vi "UE9 4-Channel Frequency Output.vi"(8 "error in":errorcluster, 10 "Timer0 Frequency [Hz]":dbl=1000.0 format="%.1f") -> (0 "error out":errorcluster, 2 "Actual Frequency 0":dbl format="%.1f")   [LabVIEW 2021]
panel:
  in  "Case Constant\n(See Context Help)":bool
  out "FreqDivisor3":u8
  out "FreqDivisor2":u8
  out "FreqDivisor1":u8
  out "FreqDivisor0":u8
  out "Actual Frequency 3":dbl format="%.1f"
  out "Actual Frequency 2":dbl format="%.1f"
  out "Actual Frequency 1":dbl format="%.1f"
  in  "Timer3 Frequency [Hz]":dbl=4000.0 format="%.1f"
  in  "Timer2 Frequency [Hz]":dbl=3000.0 format="%.1f"
  in  "Timer1 Frequency [Hz]":dbl=2000.0 format="%.1f"
  in  "FirstFound":bool=TRUE
  in  "Address":string="1"
  in  "ConnectionType":u16(ring) items=["LJ_ctUSB", "LJ_ctETHERNET"]
  in  "# of frequency outputs to enable":u32=4
  out "TimerClockDivisor":u8
  out "TimerClockConfig":string
  out "Error Message":string
  # "Demonstrates 4 channels of frequency output on FIO0-FIO3.\nAssumes Control power level is at the default level of \"High\" (Control firmware 1.08 or higher).\nA simple algorithm decides the clock settings to get the desired Timer0 frequency.  Then the\nfrequency divisor value is adjusted, as much as possible, to get the frequencies specified for\nother channels.  Because of these simple algorithms, best results will most likely occur if Timer0 is\nthe lowest frequency of the 4."
  # "Clock configuration determined\nby first channel."
  # "24 MHz max, 5.7 Hz min"
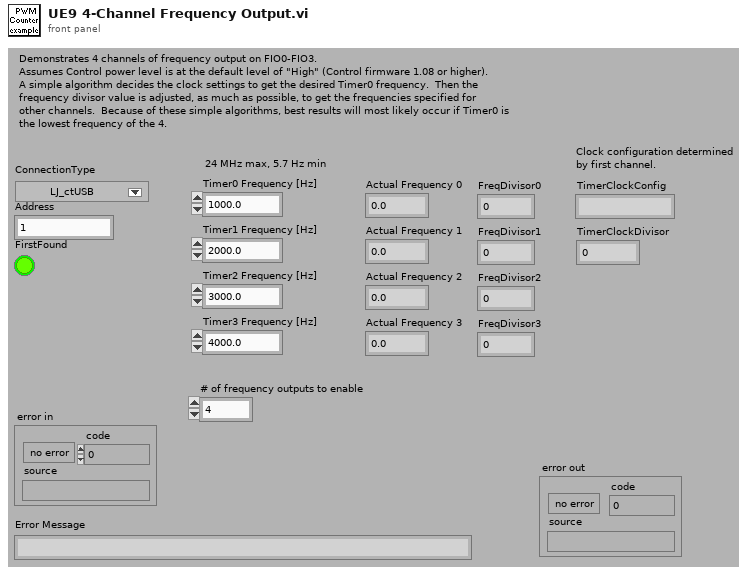
[diagram p1: front panel]
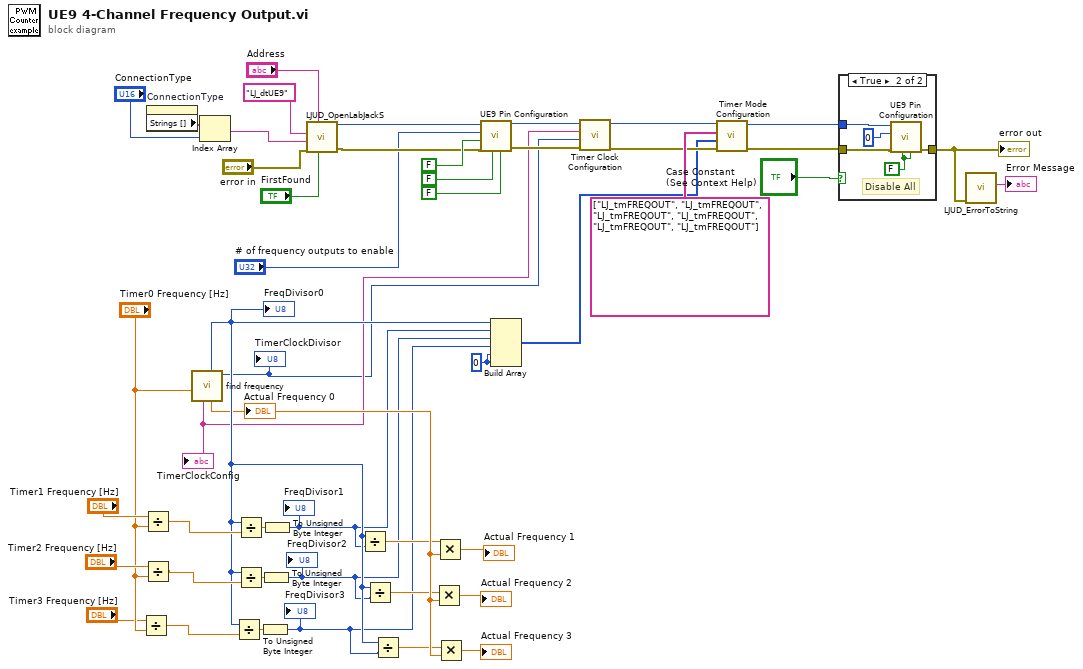
[diagram p0: block diagram]
diagram:
  w32 = 0 ("Input Element")
  n1 = Divide(x="Timer3 Frequency [Hz]", y="Timer0 Frequency [Hz]") -> (x/y=w36:dbl)
  n2 = Divide(x="Timer1 Frequency [Hz]", y="Timer0 Frequency [Hz]") -> (x/y=w38:dbl)
  n3 = Divide(x="Timer2 Frequency [Hz]", y="Timer0 Frequency [Hz]") -> (x/y=w37:dbl)
  n4 = property on="ConnectionType" class="Ring (strict)"() -> ("Strings []"=w18:string[])  [unwired: 2 in, 2 out]
  n5 = call "find frequency.vi"("target frequency"="Timer0 Frequency [Hz]") -> ("ClockDivisor"=w2:i32, "Frequency"=w30:dbl, "FreqDivisor"=w31:i32, "Clock Source"=w3:string)  [unwired: 5 in, 2 out]
  "Actual Frequency 0" <- w30
  "TimerClockConfig" <- w3
  "TimerClockDivisor" <- w2
  "FreqDivisor0" <- w31
  n6 = Index Array(array=w18, index="ConnectionType") -> (element=w17:string)
  n7 = Divide(x=w31, y=w36) -> (x/y=w34:dbl)
  n8 = Divide(x=w31, y=w38) -> (x/y=w35:dbl)
  n9 = Divide(x=w31, y=w37) -> (x/y=w33:dbl)
  n10 = To Unsigned Byte Integer(number=w34) -> (unsigned 8bit integer=w21:u8)
  "FreqDivisor3" <- w21
  n11 = To Unsigned Byte Integer(number=w33) -> (unsigned 8bit integer=w22:u8)
  "FreqDivisor2" <- w22
  n12 = To Unsigned Byte Integer(number=w35) -> (unsigned 8bit integer=w23:u8)
  "FreqDivisor1" <- w23
  n13 = call "LJUD_OpenLabJackS.vi"("FirstFound"="FirstFound", "Address"="Address", "error in"="error in", "ConnectionType"=w17, "DeviceType"="LJ_dtUE9") -> ("error out"=w7:errorcluster, "Handle"=w8:i32)  [unwired: 4 in, 1 out]
  n14 = Divide(x=w31, y=w23) -> (x/y=w29:dbl)
  n15 = Divide(x=w31, y=w22) -> (x/y=w28:dbl)
  n16 = Divide(x=w31, y=w21) -> (x/y=w27:dbl)
  n17 = Multiply(x=w28, y=w30) -> (x*y=→"Actual Frequency 2":dbl)
  n18 = Multiply(x=w29, y=w30) -> (x*y=→"Actual Frequency 1":dbl)
  n19 = Multiply(x=w27, y=w30) -> (x*y=→"Actual Frequency 3":dbl)
  n20 = call "UE9 Pin Configuration.vi"("Enable Counter1"=FALSE ("Enable Counter0"), "Enable Counter0"=FALSE, "error in"=w7, "Enable DACs"=FALSE ("Enable Counter0"), "Number of Timers Enabled"="# of frequency outputs to enable", "Handle In"=w8) -> ("error out"=w13:errorcluster, "Handle Out"=w12:i32)  [unwired: 4 in]
  n21 = Build Array(w31, w23, w22, w21, w32, w32) -> (w1:i32[])
  n22 = call "Timer Clock Configuration.vi"("error in"=w13, "Timer Clock Divisor"=w2, "Timer Clock Base"=w3, "Handle In"=w12) -> ("error out"=w14:errorcluster, "Handle Out"=w11:i32)  [unwired: 6 in]
  n23 = call "Timer Mode Configuration.vi"("error in"=w14, "TimerValues"=w1, "TimerModes"=string[] ["LJ_tmFREQOUT", "LJ_tmFREQOUT", "LJ_tmFREQOUT", "LJ_tmFREQOUT", "LJ_tmFREQOUT", "LJ_tmFREQOUT"], "Handle In"=w11) -> ("error out"=w5:errorcluster, "Handle Out"=w6:i32)  [unwired: 6 in]
  n24 = case shown="True" "Case Constant\n(See Context Help)" {
    tunnel: w5 -> [w49 w54]
    tunnel: w6 -> [_ w53]
    tunnel: [w49 w50] -> w44
    frame False {
    }
    frame True {
      w52 = FALSE ("Enable Counter0")
      # "Disable All"
      n25 = call "UE9 Pin Configuration.vi"("Enable Counter1"=w52, "Enable Counter0"=w52, "error in"=w54, "Number of Timers Enabled"=u8 0 ("# Timers Enabled"), "Handle In"=w53) -> ("error out"=w50:errorcluster)  [unwired: 5 in, 1 out]
    }
  }
  "error out" <- w44
  n26 = call "LJUD_ErrorToString.vi"("error in"=w44) -> ("String"=→"Error Message":string)  [unwired: 10 in]
